vi "Write Enable.vi"(8 "error in (no error)":errorcluster, 10 "Enable":bool, 11 "ProjectLoader in":refnum<class "ProjectLoader.lvclass">) -> (0 "error out":errorcluster, 3 "ProjectLoader out":refnum<class "ProjectLoader.lvclass">)   [LabVIEW 2015, in "ProjectLoader.lvclass"]
uses:
  ProjectLoader.lvclass
  ProjectLoader.lvclass/ProjectLoader.ctl
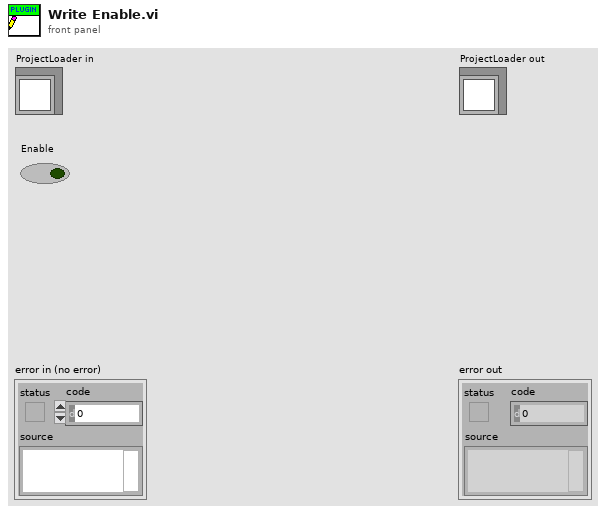
[diagram p1: front panel]
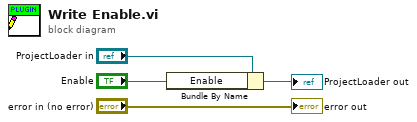
[diagram p0: block diagram]
diagram:
  n1 = Bundle By Name(cluster="ProjectLoader in", "Enable"="Enable") -> (→"ProjectLoader out":refnum<class "ProjectLoader.lvclass">)
  "error out" <- "error in (no error)"
